vi "Compare ECAT Vars.vi"(8 "Fehler (Eingang, kein Fehler)":errorcluster, 11 "I/O Output Vars (Eingang)":T1[](array[typedef]) {"VS ref" format="%.0x"}) -> (0 "Fehler (Ausgang)":errorcluster, 3 "I/O Output Vars (Ausgang)":T1[](array[typedef]) {"VS ref" format="%.0x"})   [LabVIEW 2017, in "Scan Engine Custom Device.lvlib"]
uses:
  Scan Engine Custom Device.lvlib
  Type Defs/Generic ECAT Slave IOV Cluster.ctl
  <vilib>/NI Veristand/Custom Device API/Custom Device Item Ref.ctl
  Type Defs/UDV Data Type.ctl
  Globals/Property Strings.vi
  <vilib>/NI Veristand/Custom Device API/Get Item Property (String).vi
  <vilib>/NI Veristand/Custom Device API/Get Item Property (I32).vi
  Globals/Error Strings.vi
  <vilib>/NI Veristand/Custom Device API/Custom Device API.lvlib
  <vilib>/NI Veristand/Custom Device Tools/Custom Device Utility Library/Custom Device Utility Library.lvlib
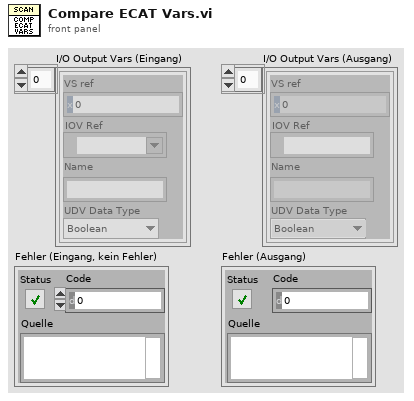
[diagram p1: front panel]
types:
  T1 = typedef "Scan Engine Custom Device.lvlib/Generic ECAT Slave IOV Cluster.ctl" = cluster{"VS ref":T2, "IOV Ref":refnum<k21>, "Name":string, "UDV Data Type":T3}
  T2 = typedef "Custom Device API.lvlib/Custom Device Item Ref.ctl" = u64
  T3 = typedef "Scan Engine Custom Device.lvlib/UDV Data Type.ctl" = enum16{"Boolean", "Fixed Point", "Int8", "Int16", "Int32", "Int64", "U32 Bit Field", "UInt8", "UInt16", "UInt32", "UInt64", "Other"}
  T4 = typedef "Custom Device API.lvlib/Custom Device Item Info.ctl" = cluster{"Name":string, "Is Channel":bool, "GUID":string, "Is Waveform":bool}
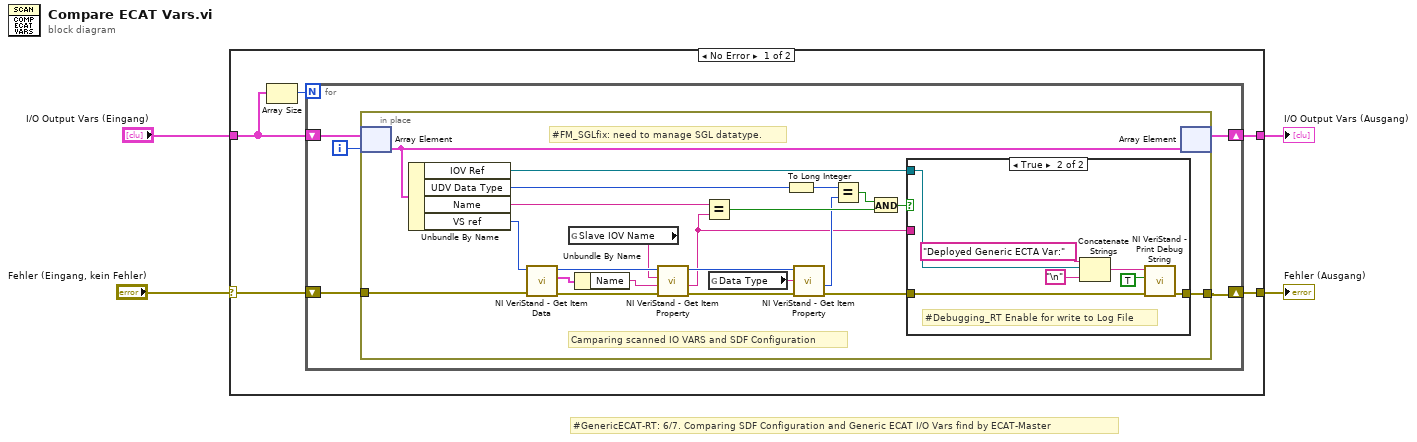
[diagram p0: block diagram]
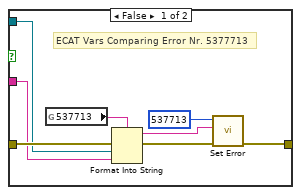
[diagram p2: hidden frame]
diagram:
  # "#GenericECAT-RT: 6/7. Comparing SDF Configuration and Generic ECAT I/O Vars find by ECAT-Master"
  n1 = case shown="No Error" "Fehler (Eingang, kein Fehler)" {
    selector: "Fehler (Eingang, kein Fehler)" -> [w6 w51]
    tunnel: [w9 w52] -> w4
    tunnel: [w5 w51] -> w3
    tunnel: "I/O Output Vars (Eingang)" -> [w8 w52]
    frame No Error {
      n2 = Array Size(array=w8) -> (size(s)=w7:i32)
      n3 = for {
        N: w7 -> [_]
        shift-right: [w10] -> w5
        shift-left: w6 -> [w12]
        shift-right: [w11] -> w9
        shift-left: w8 -> [w14]
        i -> [w13]
        n4 = in-place {
          in-place-border: w12 -> [w31]
          in-place-border: [w25] -> w10
          # "#FM_SGLfix: need to manage SGL datatype."
          # "Camparing scanned IO VARS and SDF Configuration"
          n5 = in-place-array #1(w14, w13) -> (w30:T1)
          n6 = Unbundle By Name(w30) -> ("IOV Ref"=w20:refnum<k21>, "UDV Data Type"=w22:T3, "Name"=w24:string, "VS ref"=w19:T2)
          n7 = call <vilib>:"NI VeriStand - Get Item Data.vi"("error in (no error)"=w31, "Item Ref in"=w19) -> ("error out"=w34:errorcluster, "Item Info"=w35:T4, "Item Ref out"=w33:T2)  [unwired: 6 in, 1 out]
          n8 = global read "Property Strings.vi" "Slave IOV Name"() -> (w15:string)
          n9 = Unbundle By Name(w35) -> ("Name"=w16:string)
          n10 = call-poly <vilib>:"NI VeriStand - Get Item Property.vi"("Default Value"=w16, "Property Name"=w15, "Item Ref in"=w33) -> ("Value"=w17:string, "Item Ref out"=w18:T2)  [unwired: 5 in, 2 out]
          n11 = Equal?(x=w24, y=w17) -> (x = y?=w28:bool)
          n12 = global read "Property Strings.vi" "Data Type"() -> (w32:string)
          n13 = To Long Integer(number=w22) -> (32bit integer=w21:i32)
          n14 = call-poly <vilib>:"NI VeriStand - Get Item Property.vi"("error in (no error)"=w34, "Property Name"=w32, "Item Ref in"=w18) -> ("error out"=w26:errorcluster, "Value"=w23:i32)  [unwired: 5 in, 2 out]
          n15 = Equal?(x=w21, y=w23) -> (x = y?=w29:bool)
          n16 = And(x=w29, y=w28) -> (x .and. y?=w27:bool)
          n17 = case shown="True" w27 {
            tunnel: w26 -> [w39 w50]
            tunnel: [w38 w49] -> w25
            tunnel: w20 -> [w37 w45]
            tunnel: w17 -> [w36 _]
            frame False {
              # "ECAT Vars Comparing Error Nr. 5377713"
              n18 = global read "Error Strings.vi" "537713"() -> (w40:string)
              n19 = Format Into String(format string=w40, error in=w39, w37, w36) -> (resulting string=w42:string, error out=w41:errorcluster)  [unwired: 1 in]
              n20 = call "Set Error.vi"("error in (no error)"=w41, "Message"=w42, "Code"=537713 ("error code (0)")) -> ("error out"=w38:errorcluster)  [unwired: 8 in]
            }
            frame True {
              # "#Debugging_RT Enable for write to Log File"
              n21 = Concatenate Strings("Deployed Generic ECTA Var:", w45, "\n") -> (w48:string)
              n22 = call <vilib>:"NI VeriStand - Print Debug String.vi"("error in (no error)"=w50, "Add to log file? (T)"=TRUE, "Message"=w48) -> ("error out"=w49:errorcluster)  [unwired: 8 in]
            }
          }
          n23 = in-place-array #1(w30) -> (w11:T1[])  [unwired: 1 out]
        }
      }
    }
    frame Error {
    }
  }
  "I/O Output Vars (Ausgang)" <- w4
  "Fehler (Ausgang)" <- w3
